vi "Get Channel States and Connections.vi"(8 "error in (no error)":errorcluster, 11 "Channel Ref in":T4 format="%.0x") -> (0 "error out":errorcluster, 2 "Routing Channel States":T1, 3 "Channel Ref out":T4=18446744073709551615 format="%.0x")   [LabVIEW 2017, in "SLSC Switch Scripting.lvlib"]
uses:
  SLSC Switch Scripting.lvlib
  <vilib>/NI Veristand/Custom Device API/Custom Device Item Ref.ctl
  Channel States.ctl
  Routing State.ctl
  Connection.ctl
  NationalInstruments.VeriStand.SystemDefinitionAPI
  SLSC Scripting Constants.vi
  <vilib>/NI VeriStand/Custom Device API/Custom Device API.lvlib
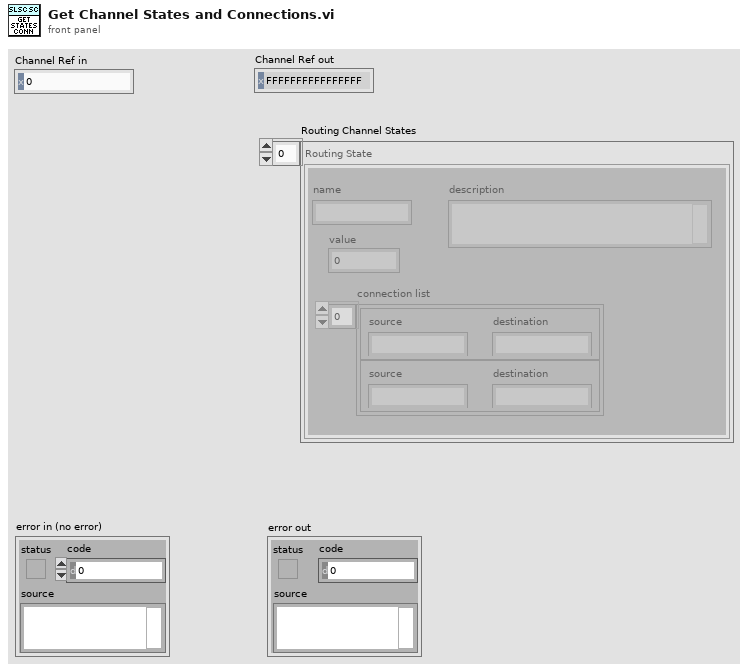
[diagram p1: front panel]
types:
  T1 = typedef "SLSC Switch Scripting.lvlib/Channel States.ctl" = T2[]
  T2 = typedef "SLSC Switch Scripting.lvlib/Routing State.ctl" = cluster{"name":string, "description":string, "value":i32, "connection list":T3[]}
  T3 = typedef "SLSC Switch Scripting.lvlib/Connection.ctl" = cluster{"source":string, "destination":string}
  T4 = typedef "Custom Device API.lvlib/Custom Device Item Ref.ctl" = u64
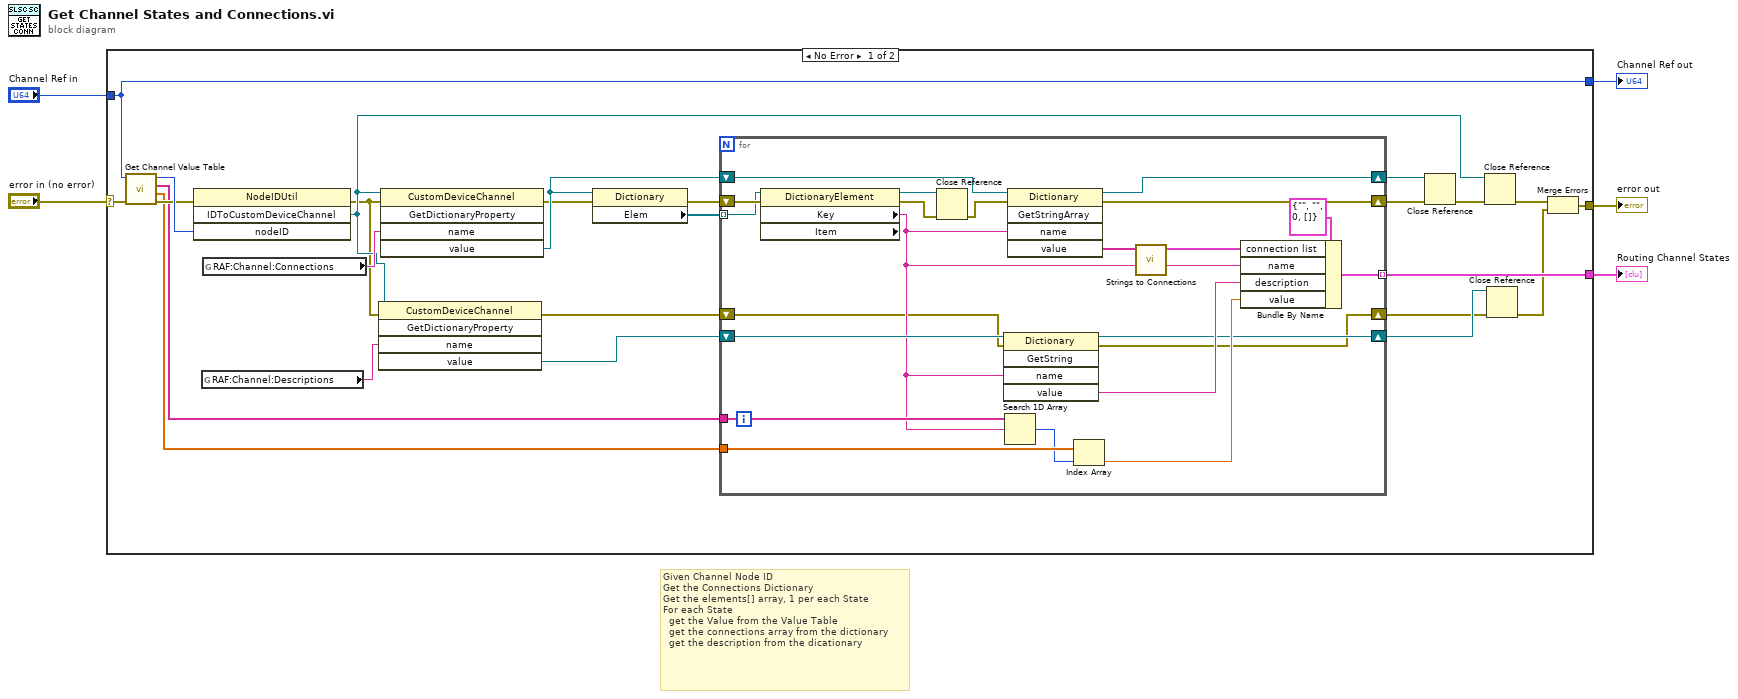
[diagram p0: block diagram]
diagram:
  # "Given Channel Node ID\nGet the Connections Dictionary\nGet the elements[] array, 1 per each State\nFor each State\n  get the Value from the Value Table\n  get the connections array from the dictionary\n  get the description from the dicationary"
  n1 = case shown="No Error" "error in (no error)" {
    selector: "error in (no error)" -> [w25 w54]
    tunnel: [w6 w54] -> w4
    tunnel: "Channel Ref in" -> [w27 w53]
    tunnel: [w27 w53] -> w2
    tunnel: [w28 _] -> w1
    frame No Error {
      n2 = call "Get Channel Value Table.vi"("error in (no error)"=w25, "Channel Ref in"=w27) -> ("error out"=w24:errorcluster, "Values"=w22:dbl[], "States"=w23:string[], "Channel Ref out"=w26:T4)  [unwired: 6 in]
      n3 = invoke class="NodeIDUtil" method="IDToCustomDeviceChannel"(error in=w24, "nodeID"=w26) -> (error out=w12:errorcluster, "IDToCustomDeviceChannel"=w15:refnum<k24>)  [unwired: 2 in, 2 out]
      n4 = global read "SLSC Scripting Constants.vi" "RAF:Channel:Descriptions"() -> (w16:string)
      n5 = global read "SLSC Scripting Constants.vi" "RAF:Channel:Connections"() -> (w19:string)
      n6 = invoke class="CustomDeviceChannel" method="GetDictionaryProperty"(reference=w15, error in=w12, "name"=w16) -> (error out=w11:errorcluster, "value"=w14:refnum<k24>)  [unwired: 2 in, 3 out]
      n7 = invoke class="CustomDeviceChannel" method="GetDictionaryProperty"(reference=w15, error in=w12, "name"=w19) -> (error out=w21:errorcluster, "value"=w29:refnum<k24>)  [unwired: 2 in, 3 out]
      n8 = property class="Dictionary"(reference=w29, error in=w21) -> (error out=w20:errorcluster, "Elem"=w17:refnum<k24>[])  [unwired: 1 out]
      n9 = for {
        shift-right: [w37] -> w30
        shift-left: w20 -> [w49]
        shift-right: [w39] -> w18
        shift-left: w29 -> [w44]
        tunnel: w17 -> [w48] mode=indexing
        tunnel: [w52] -> w28 mode=indexing
        tunnel: w23 -> [w51]
        tunnel: w22 -> [w50]
        shift-right: [w35] -> w13
        shift-left: w14 -> [w38]
        shift-right: [w31] -> w10
        shift-left: w11 -> [w32]
        n10 = property class="DictionaryElement" props=["Key", "Item"](reference=w48, error in=w49) -> (reference out=w47:refnum<k24>, error out=w46:errorcluster, "Key"=w36:string)  [unwired: 1 out]
        n11 = Close Reference(reference=w47, error in (no error)=w46) -> (error out=w45:errorcluster)
        n12 = invoke class="Dictionary" method="GetString"(reference=w38, error in=w32, "name"=w36) -> (reference out=w35:refnum<k24>, error out=w31:errorcluster, "value"=w40:string)  [unwired: 2 in, 2 out]
        n13 = Search 1D Array(1D array=w51, element=w36) -> (index of element=w42:i32)  [unwired: 1 in]
        n14 = invoke class="Dictionary" method="GetStringArray"(reference=w44, error in=w45, "name"=w36) -> (reference out=w39:refnum<k24>, error out=w37:errorcluster, "value"=w34:string[])  [unwired: 2 in, 2 out]
        n15 = Index Array(array=w50, index=w42) -> (element=w41:dbl)
        n16 = call "Strings to Connections.vi"("connection strings"=w34) -> ("connection list"=w33:T3[])  [unwired: 10 in]
        n17 = Bundle By Name(cluster=T2 {"name"="", "description"="", "value"=0, "connection list"=[]} ("Routing State"), "connection list"=w33, "name"=w36, "description"=w40, "value"=w41) -> (w52:T2)
      }
      n18 = Close Reference(reference=w18, error in (no error)=w30) -> (error out=w9:errorcluster)
      n19 = Close Reference(reference=w15, error in (no error)=w9) -> (error out=w8:errorcluster)
      n20 = Close Reference(reference=w13, error in (no error)=w10) -> (error out=w7:errorcluster)
      n21 = Merge Errors(w8, w7) -> (w6:errorcluster)
    }
    frame Error {
    }
  }
  "Channel Ref out" <- w2
  "error out" <- w4
  "Routing Channel States" <- w1
